vi "DC Name to DC_UID.vi"(11 "DC Name":string) -> (3 "DC_UID":T1)   [LabVIEW 2017]
doc: "Extract Debug Client UID from Debug Client name"
uses:
  DC_UID.ctl
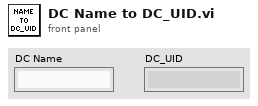
[diagram p1: front panel]
types:
  T1 = typedef "DC_UID.ctl" = string
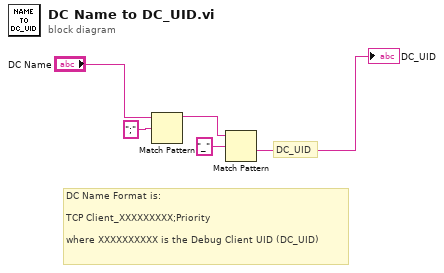
[diagram p0: block diagram]
diagram:
  # "DC Name Format is:\n\nTCP Client_XXXXXXXXX;Priority\n\nwhere XXXXXXXXXX is the Debug Client UID (DC_UID)"
  # "DC_UID"
  n1 = Match Pattern(string="DC Name", regular expression=";") -> (before substring=w3:string)  [unwired: 1 in, 3 out]
  n2 = Match Pattern(string=w3, regular expression="_") -> (after substring=→"DC_UID":string)  [unwired: 1 in, 3 out]
